vi "swap actions in sequence.vi"(6 "action index 2":i32, 7 "action index 1":i32, 8 "error in (no error)":errorcluster, 10 "sequence name":string, 11 "Simple Sequencer TBM configuration in":refnum<class "Simple Sequencer TBM configuration.lvclass">) -> (0 "error out":errorcluster, 3 "Simple Sequencer TBM configuration out":refnum<class "Simple Sequencer TBM configuration.lvclass">)   [LabVIEW 2014, in "Simple Sequencer TBM configuration.lvclass"]
doc: "Swaps the position of the two actions with the specified indices."
uses:
  Simple Sequencer TBM configuration.lvclass
  Simple Sequencer TBM configuration.lvclass/Simple Sequencer TBM configuration.ctl
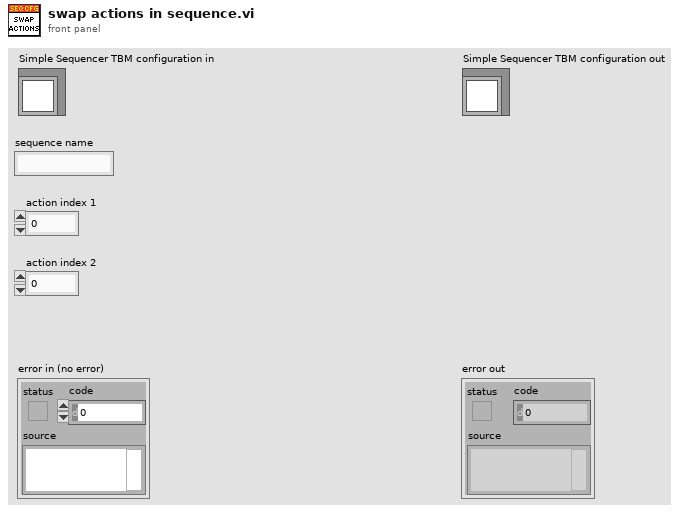
[diagram p1: front panel]
types:
  T1 = typedef "Simple Sequencer TBM configuration.lvclass/sequence definition.ctl" = cluster{"sequence name":string, "action configs":refnum<class "action configuration.lvclass">[]}
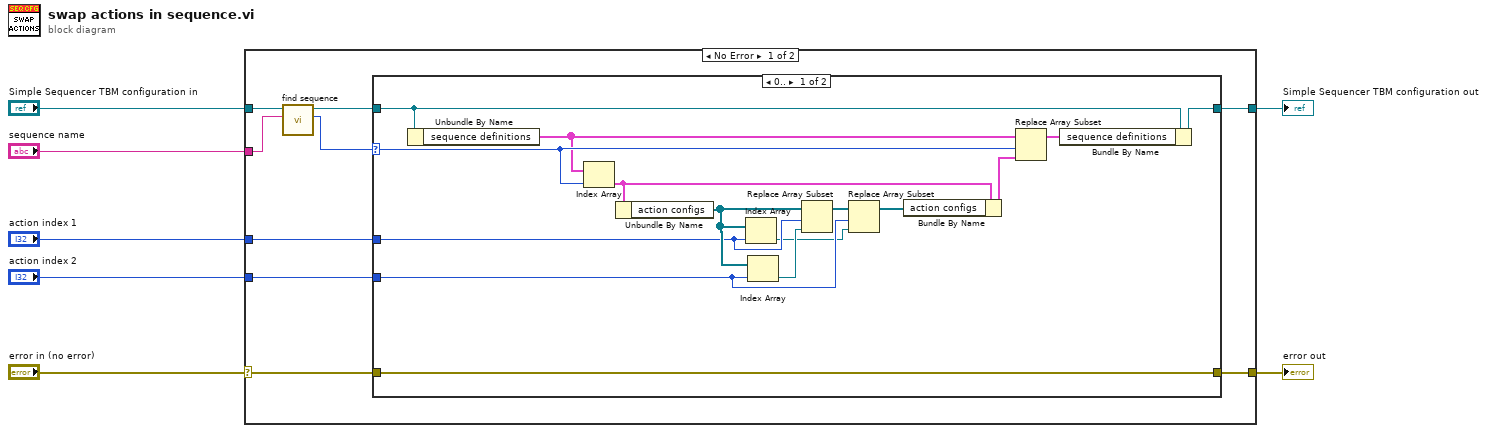
[diagram p0: block diagram]
diagram:
  n1 = case shown="No Error" "error in (no error)" {
    selector: "error in (no error)" -> [w11 w35]
    tunnel: [w12 w35] -> w6
    tunnel: [w14 w34] -> w4
    tunnel: "Simple Sequencer TBM configuration in" -> [w16 w34]
    tunnel: "sequence name" -> [w10 _]
    tunnel: "action index 1" -> [w9 _]
    tunnel: "action index 2" -> [w8 _]
    frame No Error {
      n2 = call "find sequence.vi"("sequence name"=w10, "Simple Sequencer TBM configuration in"=w16) -> ("index"=w15:i32, "Simple Sequencer TBM configuration out"=w13:refnum<class "Simple Sequencer TBM configuration.lvclass">)  [unwired: 8 in]
      n3 = case shown="0.." w15 {
        selector: w15 -> [w28 _]
        tunnel: [w29 w33] -> w14
        tunnel: w13 -> [w30 w33]
        tunnel: [w31 w32] -> w12
        tunnel: w11 -> [w31 w32]
        tunnel: w9 -> [w23 _]
        tunnel: w8 -> [w22 _]
        frame 0.. {
          n4 = Unbundle By Name(w30) -> ("sequence definitions"=w27:T1[])
          n5 = Index Array(array=w27, index=w28) -> (element=w19:T1)
          n6 = Unbundle By Name(w19) -> ("action configs"=w25:refnum<class "action configuration.lvclass">[])
          n7 = Index Array(array=w25, index=w23) -> (element=w20:refnum<class "action configuration.lvclass">)
          n8 = Index Array(array=w25, index=w22) -> (element=w21:refnum<class "action configuration.lvclass">)
          n9 = Replace Array Subset(array=w25, new element=w21, index=w23) -> (w24:refnum<class "action configuration.lvclass">[])
          n10 = Replace Array Subset(array=w24, new element=w20, index=w22) -> (w17:refnum<class "action configuration.lvclass">[])
          n11 = Bundle By Name(cluster=w19, "action configs"=w17) -> (w18:T1)
          n12 = Replace Array Subset(array=w27, new element=w18, index=w28) -> (w26:T1[])
          n13 = Bundle By Name(cluster=w30, "sequence definitions"=w26) -> (w29:refnum<class "Simple Sequencer TBM configuration.lvclass">)
        }
        frame ..-1 {
          # "#todo throw not found error"
        }
      }
    }
    frame Error {
    }
  }
  "error out" <- w6
  "Simple Sequencer TBM configuration out" <- w4
